vi "MultiScan.vi"(6 "Function":i32, 8 "error in (no error)":errorcluster caption="entrée d'erreur (pas d'erreur)", 9 "Single":bool, 11 "ExperimentIn":refnum<class "Experiment.lvclass"> caption="DNL_LabVIEW Object in") -> (0 "error out":errorcluster caption="sortie d'erreur", 1 "TimesArray":u32[](array[numeric]), 2 "ScanParsOut":dbl[](array[numeric]), 3 "ExperimentOut":refnum<class "Experiment.lvclass"> caption="DNL_LabVIEW Object out", 10 "Index":i32 caption="Index du Point" min=-15 max=15 step=1)   [LabVIEW 2019, in "Experiment.lvclass"]
uses:
  Experiment.lvclass
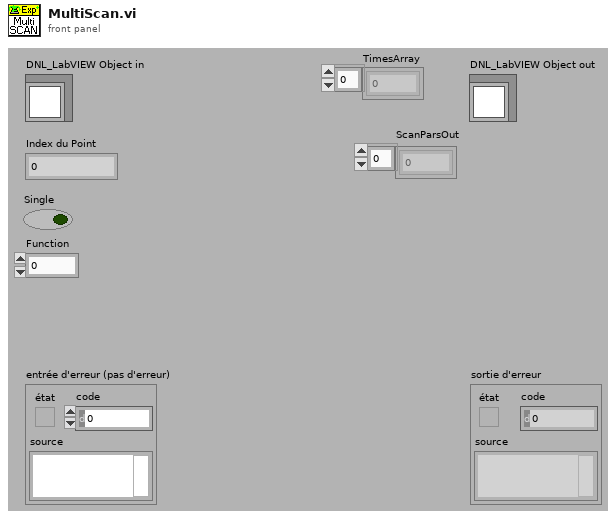
[diagram p1: front panel]
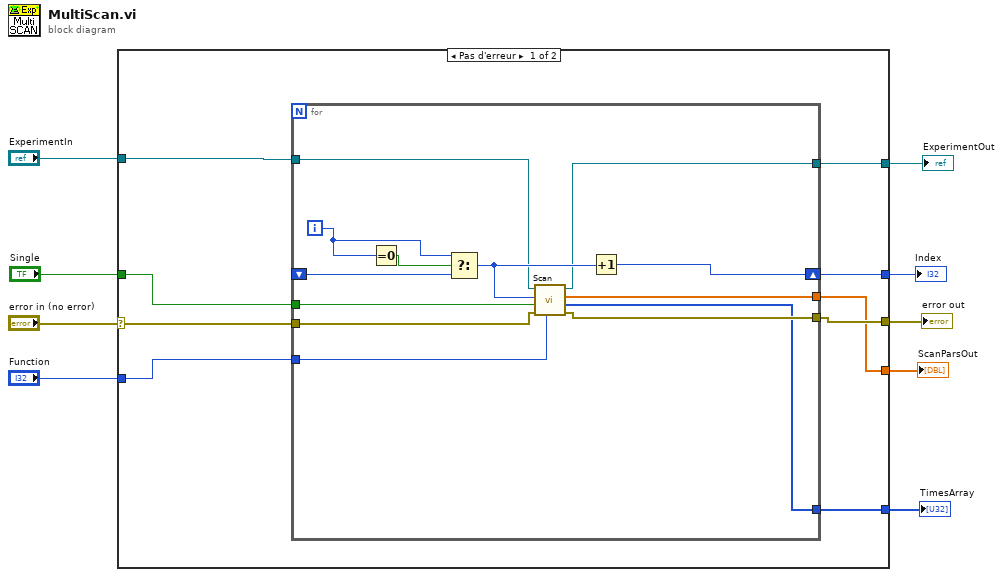
[diagram p0: block diagram]
diagram:
  n1 = case shown="Pas d'erreur" "error in (no error)" {
    selector: "error in (no error)" -> [w16 w33]
    tunnel: [w14 w33] -> w8
    tunnel: [w11 w32] -> w6
    tunnel: "ExperimentIn" -> [w15 w32]
    tunnel: "Function" -> [w17 _]
    tunnel: "Single" -> [w18 _]
    tunnel: [w13 _] -> w3
    tunnel: [w12 _] -> w2
    tunnel: [w10 _] -> w1
    frame No Error {
      n2 = for {
        tunnel: w18 -> [w31]
        shift-right: [w26] -> w13
        shift-left: _ -> [w28]
        tunnel: w17 -> [w25]
        tunnel: [w24] -> w14
        tunnel: w16 -> [w23]
        tunnel: w15 -> [w22]
        tunnel: [w21] -> w12
        tunnel: [w20] -> w11
        tunnel: [w19] -> w10
        i -> [w27]
        n3 = Equal To 0?(x=w27) -> (x = 0?=w30:bool)
        n4 = Select(t=w27, s=w30, f=w28) -> (s? t:f=w29:i32)
        n5 = call "Scan.vi"("Function"=w25, "error in (no error)"=w23, "Single"=w31, "Index"=w29, "ExperimentIn"=w22) -> ("error out"=w24:errorcluster, "TimesArray"=w21:u32[], "ScanParsOut"=w19:dbl[], "ExperimentOut"=w20:refnum<class "Experiment.lvclass">)  [unwired: 3 in]
        n6 = Increment(x=w29) -> (x+1=w26:i32)
      }
    }
    frame Error {
    }
  }
  "error out" <- w8
  "ExperimentOut" <- w6
  "Index" <- w3
  "ScanParsOut" <- w1
  "TimesArray" <- w2
